vi "SeCrTs-PPSU Feedback.vi"(7 "PPSU Queue":refnum<queue>, 8 "Error in":errorcluster, 11 "Enable PPSU":bool) -> (0 "Fehler (Ausgang)":errorcluster caption="Error out", 1 "Power":i32, 2 "Current":i32, 3 "Voltage":i32, 4 "Fault Status":bool[](array[boolean]), 5 "No .of slaves":u8)   [LabVIEW 2022 SP3]
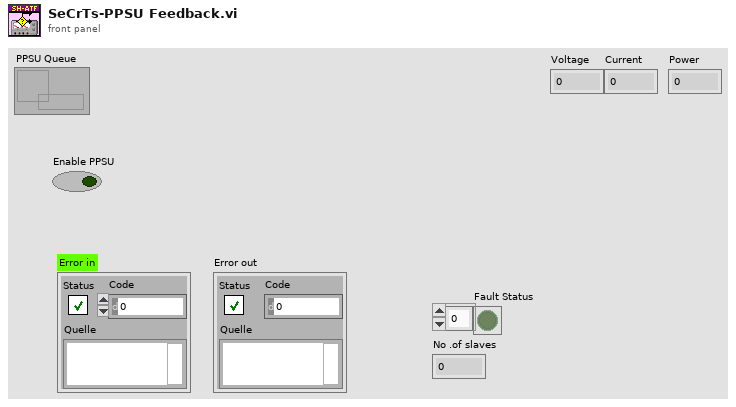
[diagram p1: front panel]
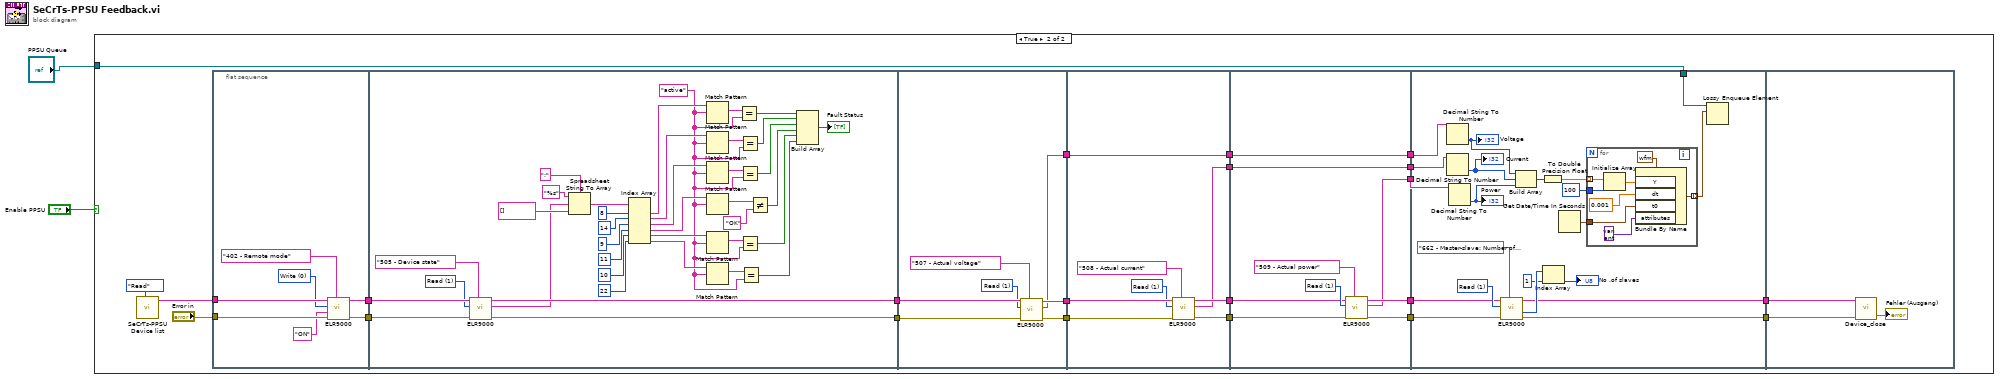
[diagram p0: block diagram]
diagram:
  n1 = case shown="True" "Enable PPSU" {
    tunnel: "PPSU Queue" -> [_ w3]
    frame False {
    }
    frame True {
      n2 = call "SeCrTs-PPSU Device list.vi"("Enum"=enum16{"Read", "Write"}."Read") -> ("Device information arrayR"=w4:string[])  [unwired: 9 in, 1 out]
      n3 = flat-sequence {
        tunnel: "Error in" -> [w31]
        tunnel: w4 -> [w30]
        tunnel: [w26] -> w24
        tunnel: [w25] -> w23
        tunnel: w24 -> [w69]
        tunnel: w23 -> [w68]
        tunnel: [w65] -> w22
        tunnel: [w64] -> w21
        tunnel: w22 -> [w76]
        tunnel: w21 -> [w75]
        tunnel: [w73] -> w20
        tunnel: [w72] -> w19
        tunnel: [w70] -> w9
        tunnel: w20 -> [w84]
        tunnel: w19 -> [w83]
        tunnel: [w80] -> w18
        tunnel: [w79] -> w17
        tunnel: [w78] -> w10
        tunnel: w9 -> [w78]
        tunnel: [w77] -> w7
        tunnel: w18 -> [w90]
        tunnel: [w88] -> w16
        tunnel: w17 -> [w91]
        tunnel: [w89] -> w15
        tunnel: [w87] -> w11
        tunnel: w10 -> [w87]
        tunnel: [w86] -> w8
        tunnel: w7 -> [w86]
        tunnel: [w85] -> w6
        tunnel: w16 -> [w112]
        tunnel: w15 -> [w111]
        tunnel: [w108] -> w14
        tunnel: [w107] -> w13
        tunnel: w11 -> [w106]
        tunnel: w8 -> [w105]
        tunnel: w6 -> [w104]
        tunnel: w3 -> [w94]
        tunnel: w14 -> [w124]
        tunnel: w13 -> [w123]
        frame #0 {
          w28 = u8 0 items=["Write", "Read"] ("Access")
          n4 = call <instrlib>:"ELR9000.vi"("Command list"="402 - Remote mode", "Error in"=w31, "Value"="ON", "Access"=w28, "Device information in"=w30) -> ("Error out"=w25:errorcluster, "Device information out"=w26:string[])  [unwired: 1 in, 2 out]
        }
        frame #1 {
          w39 = "active"
          w67 = u8 1 items=["Write", "Read"] ("Access")
          n5 = call <instrlib>:"ELR9000.vi"("Command list"="505 - Device state", "Error in"=w68, "Access"=w67, "Device information in"=w69) -> ("Error out"=w65:errorcluster, "Read data"=w62:string, "Device information out"=w64:string[])  [unwired: 2 in, 1 out]
          n6 = Spreadsheet String To Array(delimiter (Tab)=";", format string="%s", spreadsheet string=w62, array type (2D Dbl)=string[] []) -> (array=w59:string[])
          n7 = Index Array(array=w59, index #1=8 ("index"), index #2=14 ("index"), index #3=9 ("index"), index #4=11 ("index"), index #5=10 ("index"), index #6=22 ("index")) -> (element #1=w52:string, element #2=w51:string, element #3=w50:string, element #4=w49:string, element #5=w48:string, element #6=w47:string)
          n8 = Match Pattern(string=w52, regular expression=w39) -> (match substring=w46:string)  [unwired: 1 in, 3 out]
          n9 = Match Pattern(string=w51, regular expression=w39) -> (match substring=w45:string)  [unwired: 1 in, 3 out]
          n10 = Match Pattern(string=w50, regular expression=w39) -> (match substring=w44:string)  [unwired: 1 in, 3 out]
          n11 = Match Pattern(string=w49, regular expression=w39) -> (match substring=w43:string)  [unwired: 1 in, 3 out]
          n12 = Match Pattern(string=w48, regular expression=w39) -> (match substring=w41:string)  [unwired: 1 in, 3 out]
          n13 = Match Pattern(string=w47, regular expression=w39) -> (match substring=w40:string)  [unwired: 1 in, 3 out]
          n14 = Equal?(x=w46, y=w39) -> (x = y?=w38:bool)
          n15 = Equal?(x=w45, y=w39) -> (x = y?=w37:bool)
          n16 = Equal?(x=w44, y=w39) -> (x = y?=w36:bool)
          n17 = Equal?(x=w41, y=w39) -> (x = y?=w34:bool)
          n18 = Equal?(x=w40, y=w39) -> (x = y?=w33:bool)
          n19 = Not Equal?(x=w43, y="OK") -> (x != y?=w35:bool)
          n20 = Build Array(w38, w37, w36, w35, w34, w33) -> (→"Fault Status":bool[])
        }
        frame #2 {
          w74 = u8 1 items=["Write", "Read"] ("Access")
          n21 = call <instrlib>:"ELR9000.vi"("Command list"="507 - Actual voltage", "Error in"=w76, "Access"=w74, "Device information in"=w75) -> ("Error out"=w73:errorcluster, "Read data"=w70:string, "Device information out"=w72:string[])  [unwired: 2 in, 1 out]
        }
        frame #3 {
          w82 = u8 1 items=["Write", "Read"] ("Access")
          n22 = call <instrlib>:"ELR9000.vi"("Command list"="508 - Actual current", "Error in"=w84, "Access"=w82, "Device information in"=w83) -> ("Error out"=w80:errorcluster, "Read data"=w77:string, "Device information out"=w79:string[])  [unwired: 2 in, 1 out]
        }
        frame #4 {
          w93 = u8 1 items=["Write", "Read"] ("Access")
          n23 = call <instrlib>:"ELR9000.vi"("Command list"="509 - Actual power", "Error in"=w90, "Access"=w93, "Device information in"=w91) -> ("Error out"=w88:errorcluster, "Read data"=w85:string, "Device information out"=w89:string[])  [unwired: 2 in, 1 out]
        }
        frame #5 {
          w114 = u8 1 items=["Write", "Read"] ("Access")
          n24 = Decimal String To Number(string=w106) -> (number=w99:i32)  [unwired: 2 in, 1 out]
          "Voltage" <- w99
          n25 = Decimal String To Number(string=w105) -> (number=w98:i32)  [unwired: 2 in, 1 out]
          "Current" <- w98
          n26 = Decimal String To Number(string=w104) -> (number=w97:i32)  [unwired: 2 in, 1 out]
          "Power" <- w97
          n27 = call <instrlib>:"ELR9000.vi"("Command list"="662 - Master-slave: Number of initialised slaves", "Error in"=w112, "Access"=w114, "Device information in"=w111) -> ("Error out"=w107:errorcluster, "Read data (hex)"=w110:u8[], "Device information out"=w108:string[])  [unwired: 2 in, 1 out]
          n28 = Build Array(w99, w98, w97) -> (w96:i32[])
          n29 = To Double Precision Float(number=w96) -> (double precision float=w102:dbl[])
          n30 = Index Array(array=w110, index=1) -> (element=→"No .of slaves":u8)
          n31 = Get Date/Time In Seconds() -> (seconds since 1Jan1904=w100:timestamp)
          n32 = for {
            tunnel: w102 -> [w122] mode=indexing
            tunnel: 100 ("dimension size") -> [w121]
            tunnel: [w117] -> w95 mode=indexing
            tunnel: w100 -> [w115]
            n33 = Initialize Array(w122, w121) -> (w120:dbl[])
            n34 = Bundle By Name(cluster=waveform(dbl) {"t0"=timestamp(0 s since 1904-01-01), "dt"=1.0, "Y"=[]} ("waveform"), "Y"=w120, "dt"=0.001, "t0"=w115, "attributes"=variant) -> (w117:waveform(dbl))
          }
          n35 = Lossy Enqueue Element(queue=w94, element=w95) -> ()  [unwired: 1 in, 4 out]
        }
        frame #6 {
          n36 = call <instrlib>:"Device_close.vi"("error in (no error)"=w123, "Device information in"=w124) -> ("Fehler (Ausgang)"=→"Fehler (Ausgang)":errorcluster)  [unwired: 3 in]
        }
      }
    }
  }
